vi "toStringArray.vi"(8 "error in (no error)":errorcluster, 11 "PlayFile in":refnum<class "PlayFile.lvclass">) -> (0 "error out":errorcluster, 2 "eventStringArray":string[](array[string]), 3 "PlayFile out":refnum<class "PlayFile.lvclass">)   [LabVIEW 2011, in "Tools.lvlib" / "Scripting.lvlib" / "PlayFile.lvclass"]
uses:
  PlayFile.lvclass
  ScriptEvent.lvclass
  PlayFile.lvclass/PlayFile.ctl
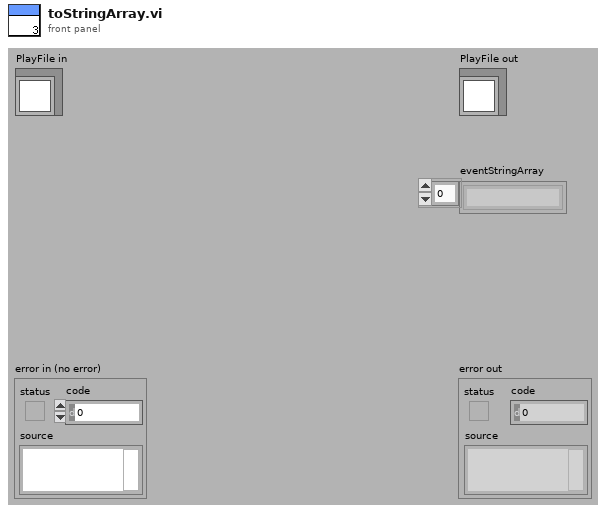
[diagram p1: front panel]
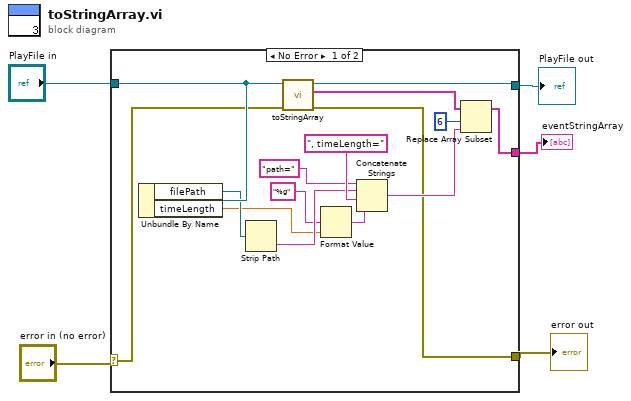
[diagram p0: block diagram]
diagram:
  n1 = case shown="No Error" "error in (no error)" {
    selector: "error in (no error)" -> [w18 w21]
    tunnel: [w13 w21] -> w4
    tunnel: [w20 w22] -> w3
    tunnel: "PlayFile in" -> [w19 w22]
    tunnel: [w14 _] -> w1
    frame No Error {
      n2 = Unbundle By Name(w19) -> ("filePath"=w11:path, "timeLength"=w7:dbl)
      n3 = Strip Path(path=w11) -> (name=w10:string)  [unwired: 1 out]
      n4 = call-parent "toStringArray.vi"("error in (no error)"=w18, "ScriptEvent in"=w19) -> ("error out"=w13:errorcluster, "eventStringArray"=w17:string[], "ScriptEvent out"=w20:refnum<class "PlayFile.lvclass">)  [unwired: 7 in]
      n5 = Format Value(format string="%g", value (0)=w7) -> (output string=w8:string)  [unwired: 1 in]
      n6 = Concatenate Strings("path=", w10, ", timeLength=", w8) -> (w15:string)
      n7 = Replace Array Subset(array=w17, new element=w15, index=6) -> (w14:string[])
    }
    frame Error {
    }
  }
  "error out" <- w4
  "PlayFile out" <- w3
  "eventStringArray" <- w1
